vi "Tosca-Purge External Recording Data.vi"(0 "Connect":T1={"Tracking"=FALSE, "Synapse"=FALSE, "Pupil"=FALSE, "Loco"=FALSE, "Retrieve"=TRUE, "Codes"=""}, 7 "Path":path=path "C:/Data/Tosca/Data/XYZ999/Session 6/XYZ999-Session6-Run19.txt", 11 "error in (no error)":errorcluster) -> (15 "error out":errorcluster={"status"=TRUE, "code"=54, "source"="TCP Open Connection in TCP-Send Command.vi:340001->Tosca-Start Synapse Recording.vi->Tosca-Start External Recording.vi->Tosca-Init Data Analysis.vi->Tosca.vi"})   [LabVIEW 2020]
uses:
  Classes/Parameters/Connect.ctl
  Classes/Parameters/Parameters.lvclass
panel:
  in  "Tracking":u16(ring)=1 caption="Tracking ready"
  in  "AI":u16(ring)=1 caption="Analog Input initializing..."
  in  "Loco":u16(ring) caption="Locomotion initializing..."
  in  "Pupil":u16(ring)=2 caption="Pupillometry initializing..."
  in  "Synapse":u16(ring)=1 caption="Synapse initializing..."
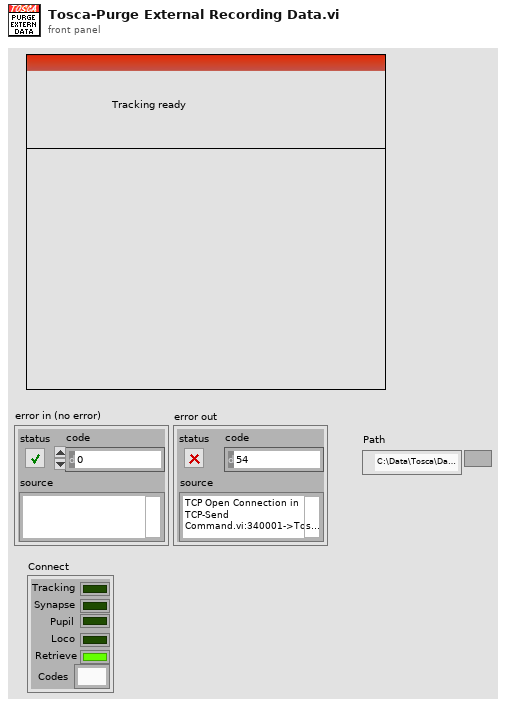
[diagram p1: front panel]
types:
  T1 = typedef "Parameters.lvclass/Connect.ctl" = cluster{"Tracking":bool, "Synapse":bool, "Pupil":bool, "Loco":bool, "Retrieve":bool, "Codes":string}
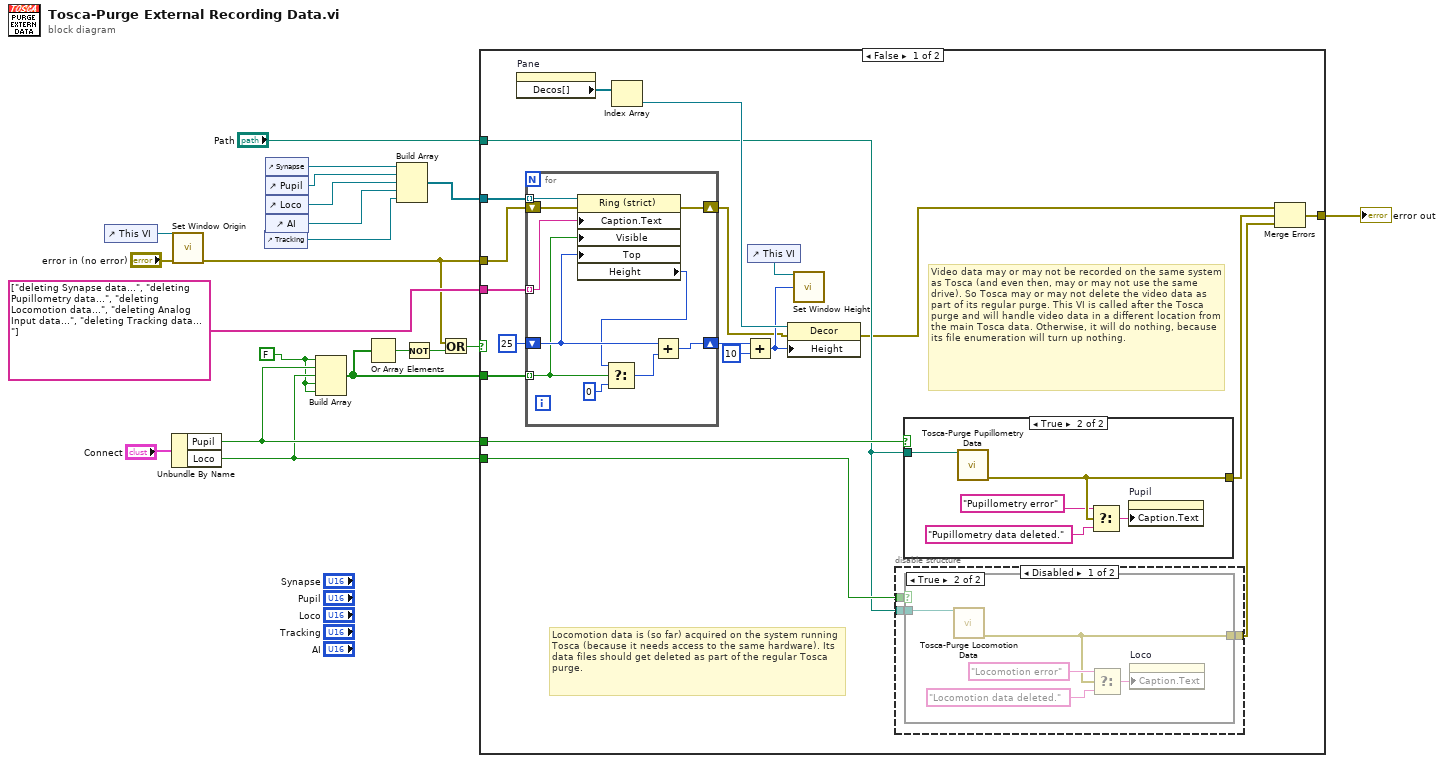
[diagram p0: block diagram]
diagram:
  w1 = FALSE
  n1 = control-ref of="This VI"() -> (w5:refnum<vi>)
  n2 = Unbundle By Name("Connect") -> ("Pupil"=w19:bool, "Loco"=w4:bool)
  n3 = call "Set Window Origin.vi"("VI in"=w5, "error in (no error)"="error in (no error)") -> ("error out"=w6:errorcluster)  [unwired: 11 in, 2 out]
  n4 = control-ref of="Tracking"() -> (w2:refnum<vi>)
  n5 = control-ref of="Synapse"() -> (w11:refnum<vi>)
  n6 = control-ref of="Pupil"() -> (w10:refnum<vi>)
  n7 = control-ref of="Loco"() -> (w8:refnum<vi>)
  n8 = control-ref of="AI"() -> (w3:refnum<vi>)
  n9 = Build Array(w1, w19, w4, w1, w1) -> (w16:bool[])
  n10 = Or Array Elements(Boolean array=w16) -> (logical OR=w17:bool)
  n11 = Build Array(w11, w10, w8, w3, w2) -> (w18:refnum<vi>[])
  n12 = Not(x=w17) -> (.not. x?=w15:bool)
  n13 = Or(x=w6, y=w15) -> (x .or. y?=w14:bool)
  n14 = case shown="False" w14 {
    tunnel: w18 -> [w39 _]
    tunnel: w6 -> [w38 w63]
    tunnel: w16 -> [w37 _]
    tunnel: [w28 w63] -> w13
    tunnel: w19 -> [w26 _]
    tunnel: "Path" -> [w23 _]
    tunnel: string[] ["deleting Synapse data...", "deleting Pupillometry data...", "deleting Locomotion data...", "deleting Analog Input data...", "deleting Tracking data..."] -> [w35 _]
    tunnel: w4 -> [w25 _]
    frame False {
      # "Video data may or may not be recorded on the same system as Tosca (and even then, may or may not use the same drive). So Tosca may or may not delete the video data as part of its regular purge. This VI is called after the Tosca purge and will handle video data in a different location from the main Tosca data. Otherwise, it will do nothing, because its file enumeration will turn up nothing."
      # "Locomotion data is (so far) acquired on the system running Tosca (because it needs access to the same hardware). Its data files should get deleted as part of the regular Tosca purge."
      n15 = property on="Pane" class="Pane"() -> ("Decos[]"=w33:refnum<vi>[])  [unwired: 2 in, 2 out]
      n16 = for {
        tunnel: w39 -> [w57] mode=indexing
        shift-right: [w55] -> w22
        shift-left: w38 -> [w56]
        tunnel: w37 -> [w50] mode=indexing
        shift-right: [w53] -> w34
        shift-left: 25 -> [w54]
        tunnel: w35 -> [w49] mode=indexing
        n17 = property class="Ring (strict)"(reference=w57, error in=w56, "Caption.Text"=w49, "Visible"=w50, "Top"=w54) -> (error out=w55:errorcluster, "Height"=w48:u32)  [unwired: 1 out]
        n18 = Select(t=w48, s=w50, f=0) -> (s? t:f=w52:u32)
        n19 = Add(x=w54, y=w52) -> (x+y=w53:u32)
      }
      n20 = Index Array(array=w33) -> (element=w32:refnum<vi>)  [unwired: 1 in]
      n21 = Add(x=w34, y=10) -> (x+y=w30:u32)
      n22 = control-ref of="This VI"() -> (w29:refnum<vi>)
      n23 = property class="Decor"(reference=w32, error in=w22, "Height"=w30) -> (error out=w21:errorcluster)  [unwired: 1 out]
      n24 = call "Set Window Height.vi"("VI in"=w29, "Height"=w30) -> ()  [unwired: 12 in, 2 out]
      n25 = disable-structure shown="Disabled" {
        disable-tunnel: w25 -> [w42 _]
        disable-tunnel: [w41 _] -> w24
        disable-tunnel: w23 -> [w40 _]
        frame Disabled {
          n26 = case shown="True" w42 {
            tunnel: [_ w43] -> w41
            tunnel: w40 -> [_ w44]
            frame False {
            }
            frame True {
              n27 = call "Tosca-Purge Locomotion Data.vi"("Path"=w44) -> ("error out"=w43:errorcluster)  [unwired: 14 in]
              n28 = Select(t="Locomotion error", s=w43, f="Locomotion data deleted.") -> (s? t:f=w45:string)
              n29 = property on="Loco" class="Ring (strict)"("Caption.Text"=w45) -> ()  [unwired: 2 in, 2 out]
            }
          }
        }
        frame Enabled {
        }
      }
      n30 = case shown="True" w26 {
        tunnel: [_ w62] -> w27
        tunnel: w23 -> [_ w58]
        frame False {
        }
        frame True {
          n31 = call "Tosca-Purge Pupillometry Data.vi"("Path"=w58) -> ("error out"=w62:errorcluster)  [unwired: 14 in]
          n32 = Select(t="Pupillometry error", s=w62, f="Pupillometry data deleted.") -> (s? t:f=w59:string)
          n33 = property on="Pupil" class="Ring (strict)"("Caption.Text"=w59) -> ()  [unwired: 2 in, 2 out]
        }
      }
      n34 = Merge Errors(w21, w27, w24) -> (w28:errorcluster)
    }
    frame True {
    }
  }
  "error out" <- w13
